vi "002 Crear random array 10 pos.vi"() -> ()   [LabVIEW 2019]
panel:
  in  "Factor d'escala":dbl
  out "nou array":dbl[](array[numeric])
  in  "nombre de posicions nou array":i32
  in  "index d'inici nou array":i32
  out "Array escalat":dbl[](array[numeric])
  out "Random array":dbl[](array[numeric])
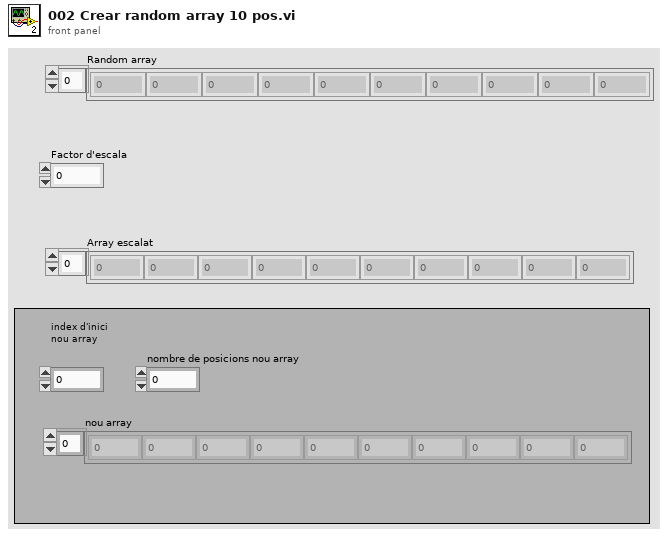
[diagram p1: front panel]
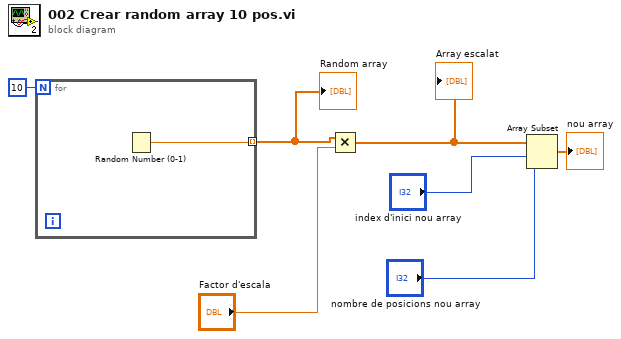
[diagram p0: block diagram]
diagram:
  n1 = for {
    N: 10 -> [_]
    tunnel: [w8] -> w6 mode=indexing
    n2 = Random Number (0-1)() -> (number: 0 to 1=w8:dbl)
  }
  "Random array" <- w6
  n3 = Multiply(x=w6, y="Factor d'escala") -> (x*y=w5:dbl[])
  "Array escalat" <- w5
  n4 = Array Subset(array=w5, index="index d'inici nou array", length="nombre de posicions nou array") -> (→"nou array":dbl[])
